vi "DisposeCore.vi"(8 "error in":errorcluster, 11 "Pizza":refnum<class "Pizza.lvclass">) -> (0 "error out":errorcluster, 3 "Pizza":refnum<class "Pizza.lvclass">)   [LabVIEW 2020, in "FactoryMethod.lvlib" / "PizzaFactoryMethod.lvlib" / "Pizza.lvclass"]
uses:
  Pizza.lvclass
  Pizza.lvclass/Pizza.ctl
  Private/TypeDef/privateDataDVR.ctl
  Private/TypeDef/privateData.ctl
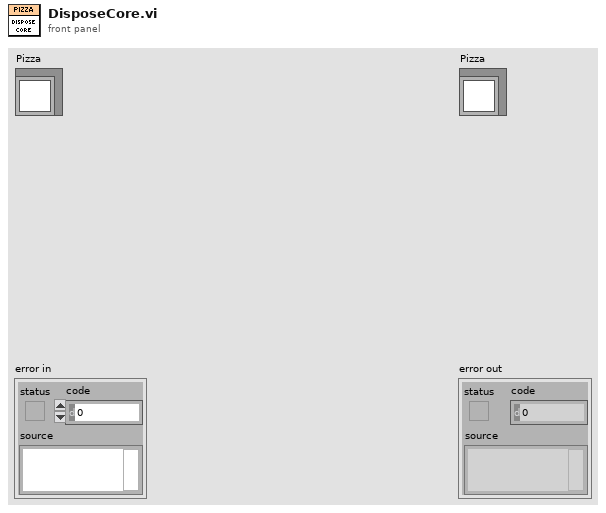
[diagram p1: front panel]
types:
  T1 = typedef "FactoryMethod.lvlib/PizzaFactoryMethod.lvlib/Pizza.lvclass/privateDataDVR.ctl" = refnum<data-value>
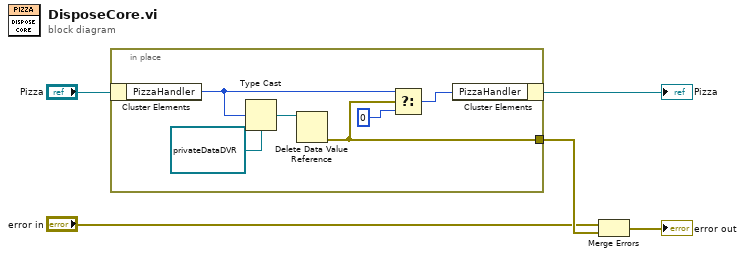
[diagram p0: block diagram]
diagram:
  n1 = in-place {
    in-place-border: [w9] -> w5
    n2 = in-place-cluster #1("Pizza") -> ("PizzaHandler"=w8:u32)
    n3 = Type Cast(type=T1 refnum ("privateDataDVR"), x=w8) -> (*(type *) &x=w11:T1)
    n4 = Delete Data Value Reference(data value reference=w11) -> (error out=w9:errorcluster)  [unwired: 1 in, 1 out]
    n5 = Select(t=w8, s=w9, f=u32 0) -> (s? t:f=w7:u32)
    n6 = in-place-cluster #1("PizzaHandler"=w7) -> (→"Pizza":refnum<class "Pizza.lvclass">)
  }
  n7 = Merge Errors("error in", w5) -> (→"error out":errorcluster)
